vi "mxwScript_Cmnd2Str_setTargetRef.vi"(8 "error in (no error)":errorcluster, 11 "data":variant) -> (0 "error out":errorcluster, 3 "outputString":string)   [LabVIEW 2020]
uses:
  codeGenAPISupport.llb/cgAPI_mxwScript_DrpTmplt_TargetRefType.ctl
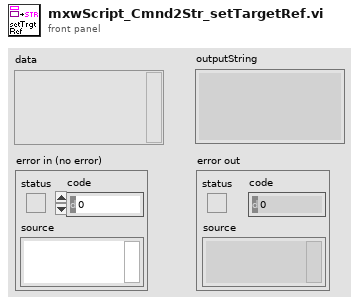
[diagram p1: front panel]
types:
  T1 = typedef "cgAPI_mxwScript_DrpTmplt_TargetRefType.ctl" = enum16{"RelativeToTemplate", "RelativeToTerminal", "AbsoluteOnRoot", "AbsoluteOnTarget", "RelativeToExistOnRoot"}
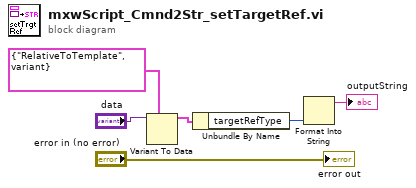
[diagram p0: block diagram]
diagram:
  n1 = Variant To Data(type=cluster{"targetRefType":T1, "data":variant} {"targetRefType"=enum."RelativeToTemplate", "data"=variant} ("targetRefData"), Variant="data") -> (data=w4:cluster{"targetRefType":T1, "data":variant})  [unwired: 1 in, 1 out]
  n2 = Unbundle By Name(w4) -> ("targetRefType"=w1:T1)
  n3 = Format Into String(w1) -> (resulting string=→"outputString":string)  [unwired: 3 in, 1 out]
  "error out" <- "error in (no error)"
